vi "Distortion_SubVI.vi"(8 "Enable":bool, 10 "Distortion level":dbl, 11 "Signal":dbl[](array[numeric])) -> (3 "Distorted Signal":dbl[](array[numeric]))   [LabVIEW 2019]
doc: "This SubVI creates distortion for the provided signal by the user. It uses \"Distrion level\" parameter that is also provided by the user. SubVI is also equipped with enable in.\n\nIN: Signal; Distortion level; Enable;\nOUT: Distorted signal;"
uses:
  <vilib>/Analysis/NI_AALPro.lvlib
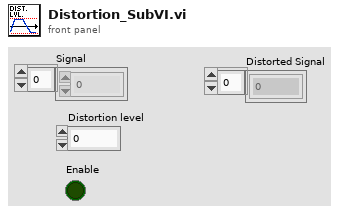
[diagram p1: front panel]
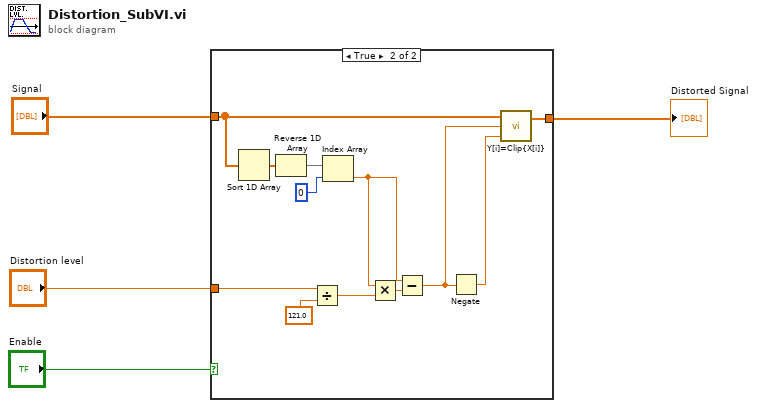
[diagram p0: block diagram]
diagram:
  n1 = case shown="True" "Enable" {
    tunnel: [w5 w17] -> w1
    tunnel: "Signal" -> [w5 w12]
    tunnel: "Distortion level" -> [_ w6]
    frame False {
    }
    frame True {
      n2 = Sort 1D Array(array=w12) -> (sorted array=w13:dbl[])
      n3 = Reverse 1D Array(array=w13) -> (reversed array=w11:dbl[])
      n4 = Divide(x=w6, y=121.0) -> (x/y=w9:dbl)
      n5 = Index Array(array=w11, index=0) -> (element=w8:dbl)
      n6 = Multiply(x=w8, y=w9) -> (x*y=w7:dbl)
      n7 = Subtract(x=w8, y=w7) -> (x-y=w14:dbl)
      n8 = Negate(x=w14) -> (-x=w16:dbl)
      n9 = call <vilib>:"Y[i]=Clip{X[i]}.vi"("lower limit"=w16, "upper limit"=w14, "Input Array"=w12) -> ("Clipped Array"=w17:dbl[])  [unwired: 1 out]
    }
  }
  "Distorted Signal" <- w1
